vi "Read Status.vi"(8 "error in (no error)":errorcluster, 11 "status pointer in":refnum<class "Status.lvclass">) -> (0 "error out":errorcluster, 2 "status":T1 {"duration" format="%d us"}, 3 "status pointer out":refnum<class "Status.lvclass">)   [LabVIEW 2017, in "DSF Core.lvlib" / "Status.lvclass"]
uses:
  Status.lvclass
  C:/Git/DSF/LabVIEW-Memory/Source/Classes/Pointer/Pointer.lvclass
  Status/Status Data.ctl
  LabVIEW-Memory/Source/Classes/Pointer/Pointer.lvclass
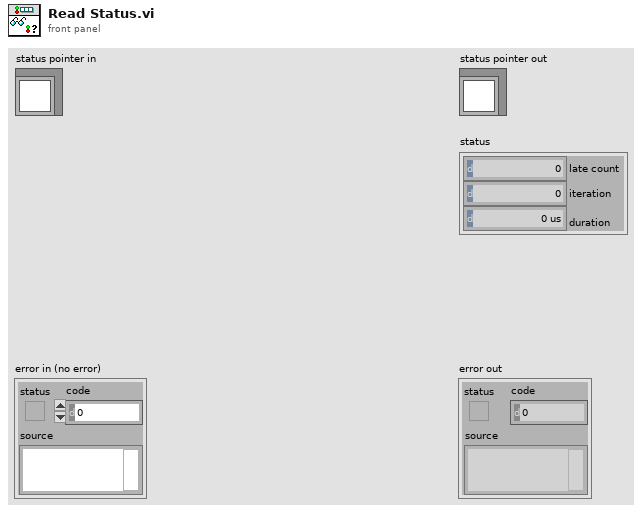
[diagram p1: front panel]
types:
  T1 = typedef "DSF Core.lvlib/Status.lvclass/Status Data.ctl" = cluster{"late count":u64, "iteration":u64, "duration":u32}
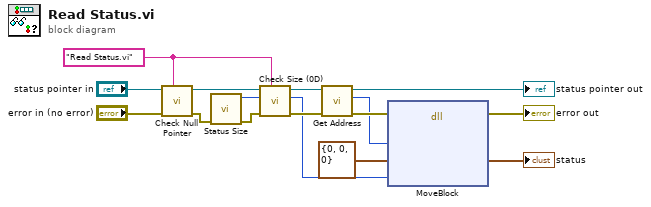
[diagram p0: block diagram]
diagram:
  w5 = "Read Status.vi" ("source vi name")
  n1 = call "Check Null Pointer.vi"("source vi name"=w5, "error in (no error)"="error in (no error)", "Pointer in"="status pointer in") -> ("error out"=w3:errorcluster, "Pointer out"=w6:refnum<class "Status.lvclass">)  [unwired: 7 in]
  n2 = call "Status Size.vi"("error in (no error)"=w3) -> ("error out"=w14:errorcluster, "size"=w2:u64)  [unwired: 9 in]
  n3 = call "Check Size (0D).vi"("source vi name"=w5, "error in (no error)"=w14, "required size"=w2, "Pointer in"=w6) -> ("error out"=w13:errorcluster, "required size out"=w1:u64, "Pointer out"=w15:refnum<class "Status.lvclass">)  [unwired: 5 in]
  n4 = call "Get Address.vi"("Pointer in"=w15) -> ("address"=w12:u64, "Pointer out"=→"status pointer out":refnum<class "Status.lvclass">)  [unwired: 9 in]
  n5 = dll-call lib="LabVIEW" fn="MoveBlock"(error in=w13, "src"=w12, "dst"=T1 {"late count"=0, "iteration"=0, "duration"=0} ("Transfer Group status"), "size"=w1) -> (error out=→"error out":errorcluster, "dst"=→"status":T1)  [unwired: 5 in, 1 out]
